vi "Configure SLSC Switch Custom Device from Switches JSON.vi"(6 "Model":string, 8 "error in":errorcluster, 9 "Resource":string, 10 "switches JSON file":path, 11 "Item Ref in":T1 format="%.0x") -> (0 "error out":errorcluster, 3 "Item Ref out":T1 format="%.0x")   [LabVIEW 2017, in "SLSC Switch Scripting.lvlib"]
uses:
  SLSC Switch Scripting.lvlib
  <vilib>/NI Veristand/Custom Device API/Custom Device Item Ref.ctl
  <vilib>/NI Veristand/Custom Device API/Custom Device API.lvlib
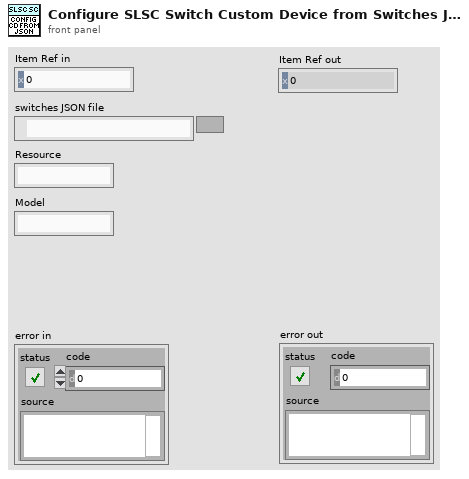
[diagram p1: front panel]
types:
  T1 = typedef "Custom Device API.lvlib/Custom Device Item Ref.ctl" = u64
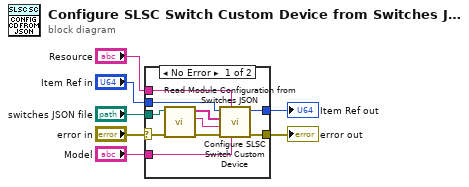
[diagram p0: block diagram]
diagram:
  n1 = case shown="No Error" "error in" {
    selector: "error in" -> [w16 w18]
    tunnel: "Item Ref in" -> [w10 w19]
    tunnel: [w14 w18] -> w4
    tunnel: [w15 w19] -> w5
    tunnel: "switches JSON file" -> [w13 _]
    tunnel: "Resource" -> [w11 _]
    tunnel: "Model" -> [w12 _]
    frame No Error {
      n2 = call "Read Module Configuration from Switches JSON.vi"("error in (no error)"=w16, "switches JSON file"=w13) -> ("error out"=w17:errorcluster, "switches json"=w8:string, "topologies"=w9:string[])  [unwired: 7 in]
      n3 = call "Configure SLSC Switch Custom Device.vi"("model"=w12, "resource"=w11, "error in (no error)"=w17, "switches json"=w8, "topologies"=w9, "SLSC Switch Custom Device Ref in"=w10) -> ("error out"=w14:errorcluster, "SLSC Switch Custom Device Ref out"=w15:T1)  [unwired: 4 in]
    }
    frame Error {
    }
  }
  "error out" <- w4
  "Item Ref out" <- w5
